vi "GNC-SET-1.vi"(0 "星敏1四元素q0":refnum<vi>, 1 "星敏1曝光时刻":refnum<vi>, 2 "星敏2四元素q3":refnum<vi>, 3 "星敏2状态字":refnum<vi>, 4 "星敏2四元素q0":refnum<vi>, 6 "星敏1四元素q2":refnum<vi>, 7 "星敏2四元素q1":refnum<vi>, 8 "星敏2曝光时刻":refnum<vi>, 9 "星敏2四元素q2":refnum<vi>, 10 "星敏1四元素q1":refnum<vi>, 11 "星敏1四元素q3":refnum<vi>, 13 "星敏1状态字":refnum<vi>) -> (14 "添加的数组":u8[](array[numeric]))   [LabVIEW 2012]
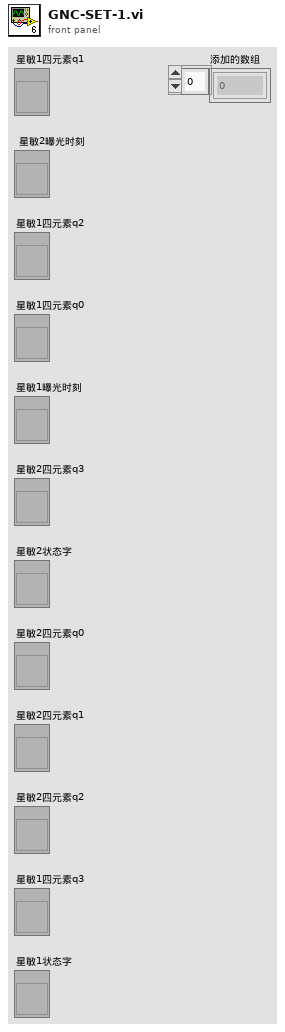
[diagram p1: front panel]
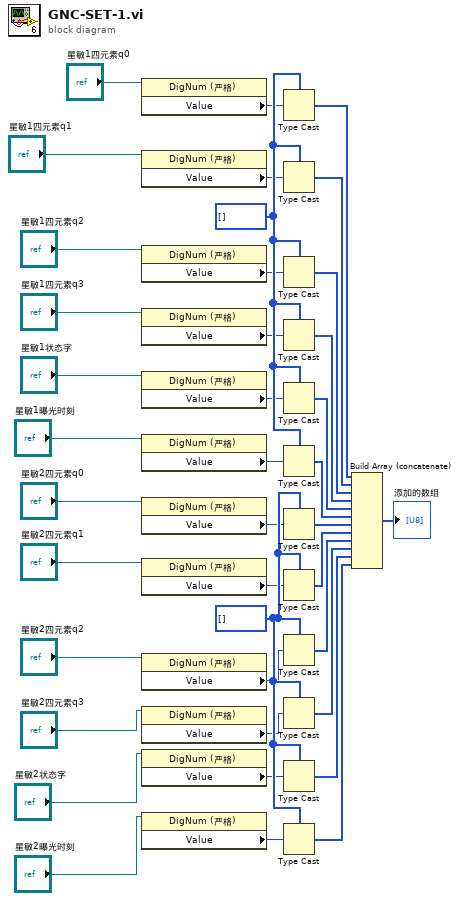
[diagram p0: block diagram]
diagram:
  w26 = u8[] []
  w25 = u8[] []
  n1 = property on="属性节点" class="DigNum (严格)"(reference="星敏1四元素q0") -> ("Value"=w13:i32)  [unwired: 1 in, 2 out]
  n2 = property on="属性节点" class="DigNum (严格)"(reference="星敏1四元素q1") -> ("Value"=w14:i32)  [unwired: 1 in, 2 out]
  n3 = property on="属性节点" class="DigNum (严格)"(reference="星敏1四元素q2") -> ("Value"=w15:i32)  [unwired: 1 in, 2 out]
  n4 = property on="属性节点" class="DigNum (严格)"(reference="星敏1四元素q3") -> ("Value"=w16:i32)  [unwired: 1 in, 2 out]
  n5 = property on="属性节点" class="DigNum (严格)"(reference="星敏1状态字") -> ("Value"=w18:i16)  [unwired: 1 in, 2 out]
  n6 = property on="属性节点" class="DigNum (严格)"(reference="星敏1曝光时刻") -> ("Value"=w17:u64)  [unwired: 1 in, 2 out]
  n7 = property on="属性节点" class="DigNum (严格)"(reference="星敏2四元素q0") -> ("Value"=w19:i32)  [unwired: 1 in, 2 out]
  n8 = property on="属性节点" class="DigNum (严格)"(reference="星敏2四元素q1") -> ("Value"=w20:i32)  [unwired: 1 in, 2 out]
  n9 = property on="属性节点" class="DigNum (严格)"(reference="星敏2四元素q2") -> ("Value"=w21:i32)  [unwired: 1 in, 2 out]
  n10 = property on="属性节点" class="DigNum (严格)"(reference="星敏2四元素q3") -> ("Value"=w22:i32)  [unwired: 1 in, 2 out]
  n11 = property on="属性节点" class="DigNum (严格)"(reference="星敏2状态字") -> ("Value"=w23:i16)  [unwired: 1 in, 2 out]
  n12 = property on="属性节点" class="DigNum (严格)"(reference="星敏2曝光时刻") -> ("Value"=w24:u64)  [unwired: 1 in, 2 out]
  n13 = Type Cast(type=w25, x=w13) -> (*(type *) &x=w27:u8[])
  n14 = Type Cast(type=w25, x=w14) -> (*(type *) &x=w28:u8[])
  n15 = Type Cast(type=w25, x=w15) -> (*(type *) &x=w29:u8[])
  n16 = Type Cast(type=w25, x=w16) -> (*(type *) &x=w30:u8[])
  n17 = Type Cast(type=w25, x=w18) -> (*(type *) &x=w31:u8[])
  n18 = Type Cast(type=w25, x=w17) -> (*(type *) &x=w32:u8[])
  n19 = Type Cast(type=w26, x=w19) -> (*(type *) &x=w33:u8[])
  n20 = Type Cast(type=w26, x=w20) -> (*(type *) &x=w34:u8[])
  n21 = Type Cast(type=w26, x=w21) -> (*(type *) &x=w35:u8[])
  n22 = Type Cast(type=w26, x=w22) -> (*(type *) &x=w36:u8[])
  n23 = Type Cast(type=w26, x=w23) -> (*(type *) &x=w37:u8[])
  n24 = Type Cast(type=w26, x=w24) -> (*(type *) &x=w38:u8[])
  n25 = Build Array (concatenate)(w27, w28, w29, w30, w31, w32, w33, w34, w35, w36, w37, w38) -> (→"添加的数组":u8[])
